vi "OEE_SCREEN_2_stations_over_cycle_time_into_cluster.vi"(6 "SCREEN_2":T1={"header_part_no"="-", "header_customer"="-", "performance_percentage"="-", "performance_target"="-", "performance_actual"="-", "OEE_target"="-", "OEE_actual"="-", "bottleneck_OP"="-", "bottleneck_target"="-", "bottleneck_actual"="-", "over_cycle_time_station_1"="-", "over_cycle_time_target_1"="-", "over_cycle_time_actual_1"="-", "over_cycle_time_station_2"="-", "over_cycle_time_target_2"="-", "over_cycle_time_actual_2"="-", "over_cycle_time_station_3"="-", "over_cycle_time_target_3"="-", "over_cycle_time_actual_3"="-", "over_cycle_time_station_4"="-", "over_cycle_time_target_4"="-", "over_cycle_time_actual_4"="-", "pace_station_1"="-", "pace_pace_1"="-", "pace_station_2"="-", "pace_pace_2"="-", "pace_station_3"="-", "pace_pace_3"="-", "pace_station_4"="-", "pace_pace_4"="-", "summary_station_1"="-", "summary_performance_1"="-", "summary_station_2"="-", "summary_performance_2"="-", "summary_station_3"="-", "summary_performance_3"="-", "summary_station_4"="-", "summary_performance_4"="-", "performance_header"="PERFORMANCE", "performance_header_target"="TARGET", "performance_header_actual"="ACTUAL", "OEE_header"="OEE", "OEE_header_target"="TARGET", "OEE_header_actual"="ACTUAL", "bottleneck_header"="LINE BOTTLENECK", "bottleneck_header_target"="TARGET", "bottleneck_header_actual"="ACTUAL", "over_cycle_time_header"="STATIONS OVER CYCLE TIME", "over_cycle_time_header_station"="STATION", "over_cycle_time_header_target"="TARGET", "over_cycle_time_header_actual"="ACTUAL", "pace_header"="OPERATIONS PACE", "pace_header_station"="STATION", "pace_header_pace"="PACE", "summary_header"="SUMMARY", "summary_header_station"="STATION", "summary_header_performance"="PERFORMANCE"}, 11 "stations_over_cycle_time":i32[][](array[numeric])) -> (4 "SCREEN_2":T1={"header_part_no"="-", "header_customer"="-", "performance_percentage"="-", "performance_target"="-", "performance_actual"="-", "OEE_target"="-", "OEE_actual"="-", "bottleneck_OP"="-", "bottleneck_target"="-", "bottleneck_actual"="-", "over_cycle_time_station_1"="-", "over_cycle_time_target_1"="-", "over_cycle_time_actual_1"="-", "over_cycle_time_station_2"="-", "over_cycle_time_target_2"="-", "over_cycle_time_actual_2"="-", "over_cycle_time_station_3"="-", "over_cycle_time_target_3"="-", "over_cycle_time_actual_3"="-", "over_cycle_time_station_4"="-", "over_cycle_time_target_4"="-", "over_cycle_time_actual_4"="-", "pace_station_1"="-", "pace_pace_1"="-", "pace_station_2"="-", "pace_pace_2"="-", "pace_station_3"="-", "pace_pace_3"="-", "pace_station_4"="-", "pace_pace_4"="-", "summary_station_1"="-", "summary_performance_1"="-", "summary_station_2"="-", "summary_performance_2"="-", "summary_station_3"="-", "summary_performance_3"="-", "summary_station_4"="-", "summary_performance_4"="-", "performance_header"="PERFORMANCE", "performance_header_target"="TARGET", "performance_header_actual"="ACTUAL", "OEE_header"="OEE", "OEE_header_target"="TARGET", "OEE_header_actual"="ACTUAL", "bottleneck_header"="LINE BOTTLENECK", "bottleneck_header_target"="TARGET", "bottleneck_header_actual"="ACTUAL", "over_cycle_time_header"="STATIONS OVER CYCLE TIME", "over_cycle_time_header_station"="STATION", "over_cycle_time_header_target"="TARGET", "over_cycle_time_header_actual"="ACTUAL", "pace_header"="OPERATIONS PACE", "pace_header_station"="STATION", "pace_header_pace"="PACE", "summary_header"="SUMMARY", "summary_header_station"="STATION", "summary_header_performance"="PERFORMANCE"})   [LabVIEW 2019]
uses:
  typedef/SCREEN_2.ctl
panel:
  # "Performance Data Output Board #2"
  # "Performance Data Output Board #2"
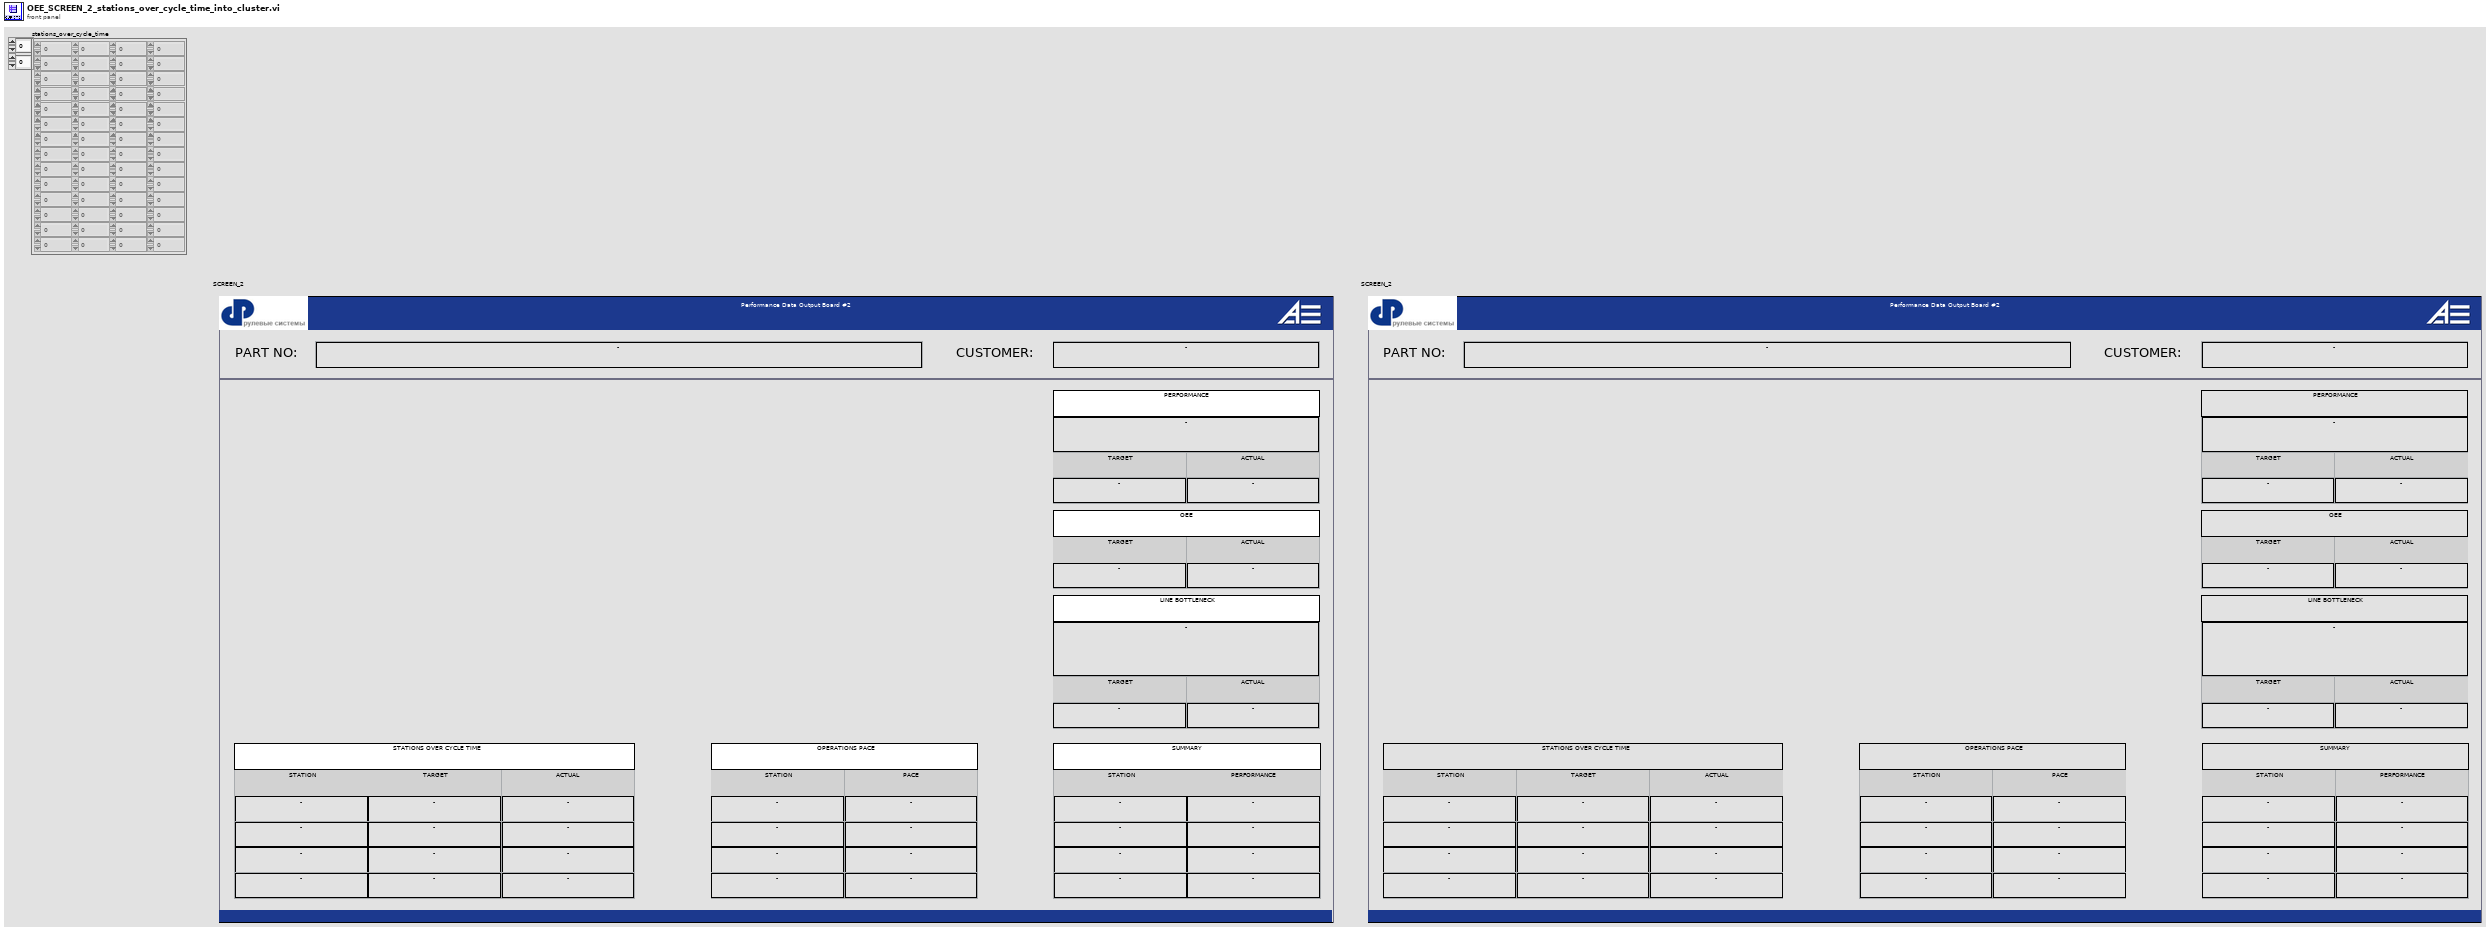
[diagram p1: front panel]
types:
  T1 = typedef "SCREEN_2.ctl" = cluster{"header_part_no":string, "header_customer":string, "performance_percentage":string, "performance_target":string, "performance_actual":string, "OEE_target":string, "OEE_actual":string, "bottleneck_OP":string, "bottleneck_target":string, "bottleneck_actual":string, "over_cycle_time_station_1":string, "over_cycle_time_target_1":string, "over_cycle_time_actual_1":string, "over_cycle_time_station_2":string, "over_cycle_time_target_2":string, "over_cycle_time_actual_2":string, "over_cycle_time_station_3":string, "over_cycle_time_target_3":string, "over_cycle_time_actual_3":string, "over_cycle_time_station_4":string, "over_cycle_time_target_4":string, "over_cycle_time_actual_4":string, "pace_station_1":string, "pace_pace_1":string, "pace_station_2":string, "pace_pace_2":string, "pace_station_3":string, "pace_pace_3":string, "pace_station_4":string, "pace_pace_4":string, "summary_station_1":string, "summary_performance_1":string, "summary_station_2":string, "summary_performance_2":string, "summary_station_3":string, "summary_performance_3":string, "summary_station_4":string, "summary_performance_4":string, "performance_header":string, "performance_header_target":string, "performance_header_actual":string, "OEE_header":string, "OEE_header_target":string, "OEE_header_actual":string, "bottleneck_header":string, "bottleneck_header_target":string, "bottleneck_header_actual":string, "over_cycle_time_header":string, "over_cycle_time_header_station":string, "over_cycle_time_header_target":string, "over_cycle_time_header_actual":string, "pace_header":string, "pace_header_station":string, "pace_header_pace":string, "summary_header":string, "summary_header_station":string, "summary_header_performance":string}
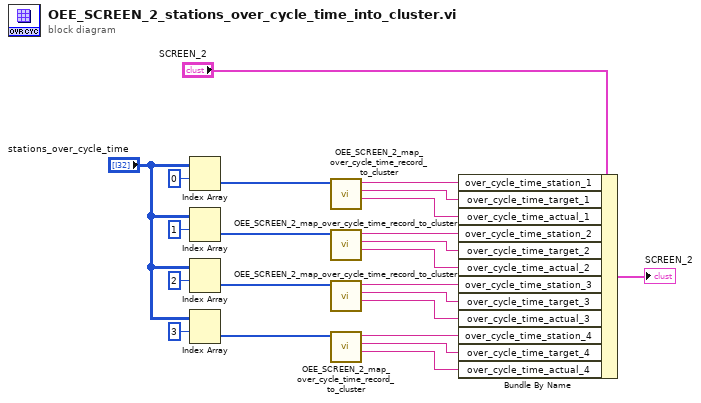
[diagram p0: block diagram]
diagram:
  n1 = Index Array(array="stations_over_cycle_time", index (row)=0) -> (element=w17:i32[])  [unwired: 1 in]
  n2 = Index Array(array="stations_over_cycle_time", index (row)=1) -> (element=w12:i32[])  [unwired: 1 in]
  n3 = Index Array(array="stations_over_cycle_time", index (row)=2) -> (element=w11:i32[])  [unwired: 1 in]
  n4 = Index Array(array="stations_over_cycle_time", index (row)=3) -> (element=w10:i32[])  [unwired: 1 in]
  n5 = call "OEE_SCREEN_2_map_over_cycle_time_record_to_cluster.vi"("stations_over_cycle_time"=w17) -> ("actual"=w14:string, "target"=w15:string, "station"=w16:string)  [unwired: 8 in]
  n6 = call "OEE_SCREEN_2_map_over_cycle_time_record_to_cluster.vi"("stations_over_cycle_time"=w12) -> ("actual"=w7:string, "target"=w8:string, "station"=w9:string)  [unwired: 8 in]
  n7 = call "OEE_SCREEN_2_map_over_cycle_time_record_to_cluster.vi"("stations_over_cycle_time"=w11) -> ("actual"=w4:string, "target"=w5:string, "station"=w6:string)  [unwired: 8 in]
  n8 = call "OEE_SCREEN_2_map_over_cycle_time_record_to_cluster.vi"("stations_over_cycle_time"=w10) -> ("actual"=w1:string, "target"=w2:string, "station"=w3:string)  [unwired: 8 in]
  n9 = Bundle By Name(cluster="SCREEN_2", "over_cycle_time_station_1"=w16, "over_cycle_time_target_1"=w15, "over_cycle_time_actual_1"=w14, "over_cycle_time_station_2"=w9, "over_cycle_time_target_2"=w8, "over_cycle_time_actual_2"=w7, "over_cycle_time_station_3"=w6, "over_cycle_time_target_3"=w5, "over_cycle_time_actual_3"=w4, "over_cycle_time_station_4"=w3, "over_cycle_time_target_4"=w2, "over_cycle_time_actual_4"=w1) -> (→"SCREEN_2":T1)
